vi "Read.vi"(8 "error in (no error)":errorcluster, 11 "Add in":refnum<class "AbsComp_One Term_U8.lvclass">) -> (0 "error out":errorcluster, 2 "Result":bool, 3 "Add out":refnum<class "AbsComp_One Term_U8.lvclass">)   [LabVIEW 2021, in "AbsComp_One Term_U8.lvclass"]
uses:
  AbsComp_One Term_U8.lvclass
  AbsComp_One Term_U8.lvclass/AbsComp_One Term_U8.ctl
  Abs_Types/U8 Integer/Abs_U8 Integer.lvclass
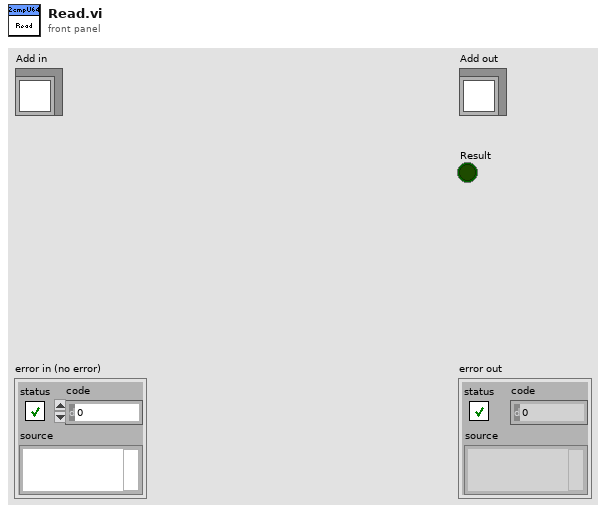
[diagram p1: front panel]
types:
  T1 = typedef "AbsComp_One Term_U8.lvclass/Abstract Type.ctl" = refnum<class "Abs_U8 Integer.lvclass">
  T2 = typedef "Abs_U8 Integer.lvclass/Type.ctl" = u8
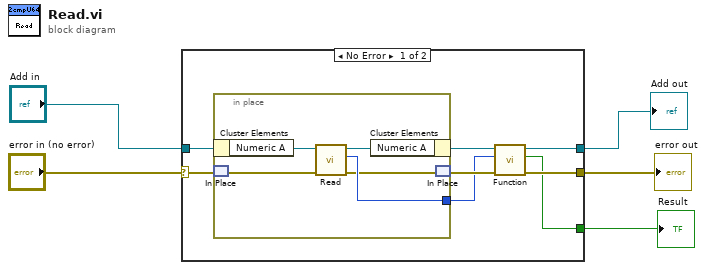
[diagram p0: block diagram]
diagram:
  n1 = case shown="No Error" "error in (no error)" {
    selector: "error in (no error)" -> [w12 w19]
    tunnel: "Add in" -> [w13 w20]
    tunnel: [w9 w20] -> w3
    tunnel: [w8 w19] -> w2
    tunnel: [w6 _] -> w1
    frame No Error {
      n2 = in-place "In Place Element Structure" {
        in-place-border: [w15] -> w7
        n3 = in-place-cluster #1(w13) -> ("Numeric A"=w18:T1)
        n4 = in-place-match #2(w12) -> (w17:errorcluster)
        n5 = call-dynamic "Read.vi"("error in (no error)"=w17, "Double Float.lvclass_340760 in"=w18) -> ("error out"=w14:errorcluster, "Value"=w15:T2, "Double Float.lvclass_340760 out"=w16:T1)  [unwired: 7 in]
        n6 = in-place-cluster #1("Numeric A"=w16) -> (w10:refnum<class "AbsComp_One Term_U8.lvclass">)
        n7 = in-place-match #2(w14) -> (w11:errorcluster)
      }
      n8 = call-dynamic "Function.vi"("error in (no error)"=w11, "Numeric"=w7, "Two Terminal in"=w10) -> ("error out"=w8:errorcluster, "Result"=w6:bool, "Two Terminal out"=w9:refnum<class "AbsComp_One Term_U8.lvclass">)  [unwired: 6 in]
    }
    frame Error {
    }
  }
  "error out" <- w2
  "Add out" <- w3
  "Result" <- w1
